vi "Top_Level_Control_1SDI_v00.vi"() -> ()   [LabVIEW 2013]
uses:
  Strict Type Defs/1BS3HD Control GUI HD.ctl
  Strict Type Defs/PII Gains.ctl
  Strict Type Defs/I16 white control.ctl
  Strict Type Defs/Thresh slider.ctl
  Strict Type Defs/Lock or Hold.ctl
  Strict Type Defs/Scan Freq Slider.ctl
  Strict Type Defs/Gains negative horizontal.ctl
  Strict Type Defs/Slider and display.ctl
  Strict Type Defs/theta 1SDI.ctl
  Strict Type Defs/1BS3HD Control GUI EPR.ctl
  Strict Type Defs/1BS3HD Lock Select.ctl
  Strict Type Defs/Scope and Safety.ctl
  Strict Type Defs/Hold All.ctl
  <vilib>/userdefined/High Color/nirio_resource_hc.ctl
  Strict Type Defs/1BS3HD Extras.ctl
  Strict Type Defs/1BS3HD Double control.ctl
  Strict Type Defs/1BS3HD I16 Control.ctl
  <vilib>/FPGAPlugInAG/PXI-7852R/niLvFpga_Open_PXI-7852R.vi
  <vilib>/rvi/interface/common/dynamic/niFpgaDynamicAddResources.vi
  <vilib>/rvi/interface/common/niFpgaWaitOnOcc.vi
  <vilib>/Utility/error.llb/Error Cluster From Error Code.vi
  <vilib>/rvi/errors/niLvFpgaAdjustHostInterfaceError.vi
  <vilib>/FPGAPlugInAG/Dynamic/niLvFpga_Close_Dynamic.vi
  <vilib>/rvi/interface/nirviOpenFPGA/nirviOpenFPGA.xnode
  FPGA Bitfiles/PI-state-4-phase_FPGATarget_3HD1BSFPGAv00_skdKazwPNYA.lvbitx
  <vilib>/rvi/interface/nirviReadWriteControl/nirviReadWriteControl.xnode
  <vilib>/rvi/interface/nirviMethod/nirviMethod.xnode
  <vilib>/rvi/interface/nirviCloseFPGA/nirviCloseFPGA.xnode
  <vilib>/rvi/interface/Simulation/niFpgaSimulationCallBeginRW.vi
  NiFpgaLv.dll
  <vilib>/FPGAPlugInAG/Dynamic/niLvFpga_ReadFifo_Dynamic.vi
  <vilib>/rvi/errors/niLvFpgaMergeErrorWithErrorCode.vi
panel:
  in  "watertank":bool
  out "Water Tank":dbl(slide)=nan scale=-0.3..0.3
  out "Top Loop Count":i32=219749
  in  "stop":bool
  in  "Hold All":T1
  in  "Extra Controls":enum32{"Scope", "Extra Controls", "X-Y Resurge"}(tab)=enum."X-Y Resurge"
  in  "Scope+Safety":T2={"Safety First"={"lim reset"=FALSE, "no limit"=FALSE, "pos slew rate * dt"=240, "neg slew rate * dt"=-240, "Count(Ticks)"=0}, "Scope IPs"={"Trigger Direction"=enum."minus-plus", "Trigger Delay (ms)"=0.0, "Aquisition Rate (kHz)"=4000.0, "Trigger Offset (V)"=0.0, "Scale Offset"={"Scaling"={"Error signal"=1, "Output"=0, "DC Monitor"=1, "Threshold"=1}, "Offset"={"Error Signal"=0, "Output"=0, "DC Monitor"=0, "Threshold"=0}}}}
  in  "Extras 1SDI":T3={"Error Bit Shift "={"EPR BS"=-1, "HD A x"=-3, "HD A p"=-3, "HD B x"=-3, "HD B p"=-3, "HD C x"=-3, "HD C p"=-3}, "I Max value"=200000, "Scan Offset"={"EPR BS"=0.0, "HD A"=1000.0, "HD B"=0.0, "HD C"=0.0}, "Scan Ampl.\n     (mV)"={"EPR BS"=5000.0, "HD A"=5000.0, "HD B"=5000.0, "HD C"=5000.0}, "Scan-PII thresh"={"EPR BS"=100, "Homodyne A"=100, "Homodyne B"=100, "Homodyne C"=100}, "Re-Scan thresh"={"EPR BS"=1, "Homodyne A"=10, "Homodyne B"=1, "Homodyne C"=0}, "Post-Offset"={"HD A x"=0.0, "HD A p"=0.0, "HD B x"=0.0, "HD B p"=0.0, "HD C x"=0.0, "HD C p"=0.0}}
  out "Graph error":errorcluster
  in  "Number of Elements":u32=4095
  in  "1SDI_FPGA_v00":T6="RIO0" caption="RIO Device"
  out "xy HD A":cluster{i16[], i16[]}(graph)
  in  "XY HD 12 ON":bool
  out "xy HD B":cluster{i16[], i16[]}(graph)
  out "xy HD B 2":cluster{i16[], i16[]}(graph)
  in  "XY HD 3 ON":bool
  in  "Scope":T7=TRUE
  out "Scope Graph":cluster{dbl[], dbl[]}[](graph)
  in  "Lock Select":T8
  in  "EPR BS":T9={"Offset Error"=-0.0003389830508474583, "Gain Error"=1, "P Gain"=16, "P Bit Shift"=-4, "I Bit Shift"=-5, "I Gain"=14, "Lock Threshold"=7, "Lock"=FALSE, "Hold"=FALSE, "Scan Frequency"=30, "Scan Bit Shift"=-7, "Gains +/- "=TRUE, "Pre- Offset Error"=0.0077966101694915265} {"Pre- Offset Error" scale=-0.01..0.02 scale format="%#_5f"; "Scan Frequency" scale=1.0..30.0; "I Gain" scale=0.0..50.0; "P Gain" scale=0.0..50.0; "Offset Error" scale=-0.02..0.02 scale format="%#_5f"}
  in  "Homodyne A":T16={"P Gain"=15, "P Bit Shift"=-4, "I Bit Shift"=-6, "I Gain"=19, "Lock Threshold"=19, "Lock"=FALSE, "Hold"=FALSE, "Scan Frequency"=11, "Scan Bit Shift"=-5, "Gains +/- "=TRUE, "Pre- Offset x"=0.008870056497175142, "Pre-Offset p"=0.0011864406779661, "Gain Error x"=3, "Lock Angle"=90.0, "Gain Error p\n\n"=7} {"Lock Angle" min=-90.0 max=90.0 scale=-90.0..90.0 scale format="%#_2g"; "Pre-Offset p" scale=-0.01..0.01 scale format="%#_5f"; "Pre- Offset x" scale=-0.03..0.05 scale format="%#_5f"; "Scan Frequency" scale=1.0..30.0; "I Gain" scale=0.0..50.0; "P Gain" scale=0.0..50.0}
  in  "Homodyne B":T16={"P Gain"=15, "P Bit Shift"=-6, "I Bit Shift"=-7, "I Gain"=21, "Lock Threshold"=16, "Lock"=FALSE, "Hold"=FALSE, "Scan Frequency"=11, "Scan Bit Shift"=-5, "Gains +/- "=TRUE, "Pre- Offset x"=-0.007062146892655368, "Pre-Offset p"=-0.0018644067796610183, "Gain Error x"=2, "Lock Angle"=0.0, "Gain Error p\n\n"=7} {"Lock Angle" min=-90.0 max=90.0 scale=-90.0..90.0 scale format="%#_2g"; "Pre-Offset p" scale=-0.03..0.03 scale format="%#_5f"; "Pre- Offset x" scale=-0.05..0.05 scale format="%#_5f"; "Scan Frequency" scale=1.0..30.0; "I Gain" scale=0.0..50.0; "P Gain" scale=0.0..50.0}
  in  "Homodyne C":T16={"P Gain"=19, "P Bit Shift"=-6, "I Bit Shift"=-7, "I Gain"=17, "Lock Threshold"=16, "Lock"=FALSE, "Hold"=FALSE, "Scan Frequency"=13, "Scan Bit Shift"=-5, "Gains +/- "=TRUE, "Pre- Offset x"=0.01327683615819209, "Pre-Offset p"=0.007627118644067794, "Gain Error x"=2, "Lock Angle"=90.0, "Gain Error p\n\n"=5} {"Lock Angle" min=-90.0 max=90.0 scale=-90.0..90.0 scale format="%#_2g"; "Pre-Offset p" scale=-0.03..0.03 scale format="%#_5f"; "Pre- Offset x" scale=-0.05..0.05 scale format="%#_5f"; "Scan Frequency" scale=1.0..30.0; "I Gain" scale=0.0..50.0; "P Gain" scale=0.0..50.0}
  # "Error Signal"
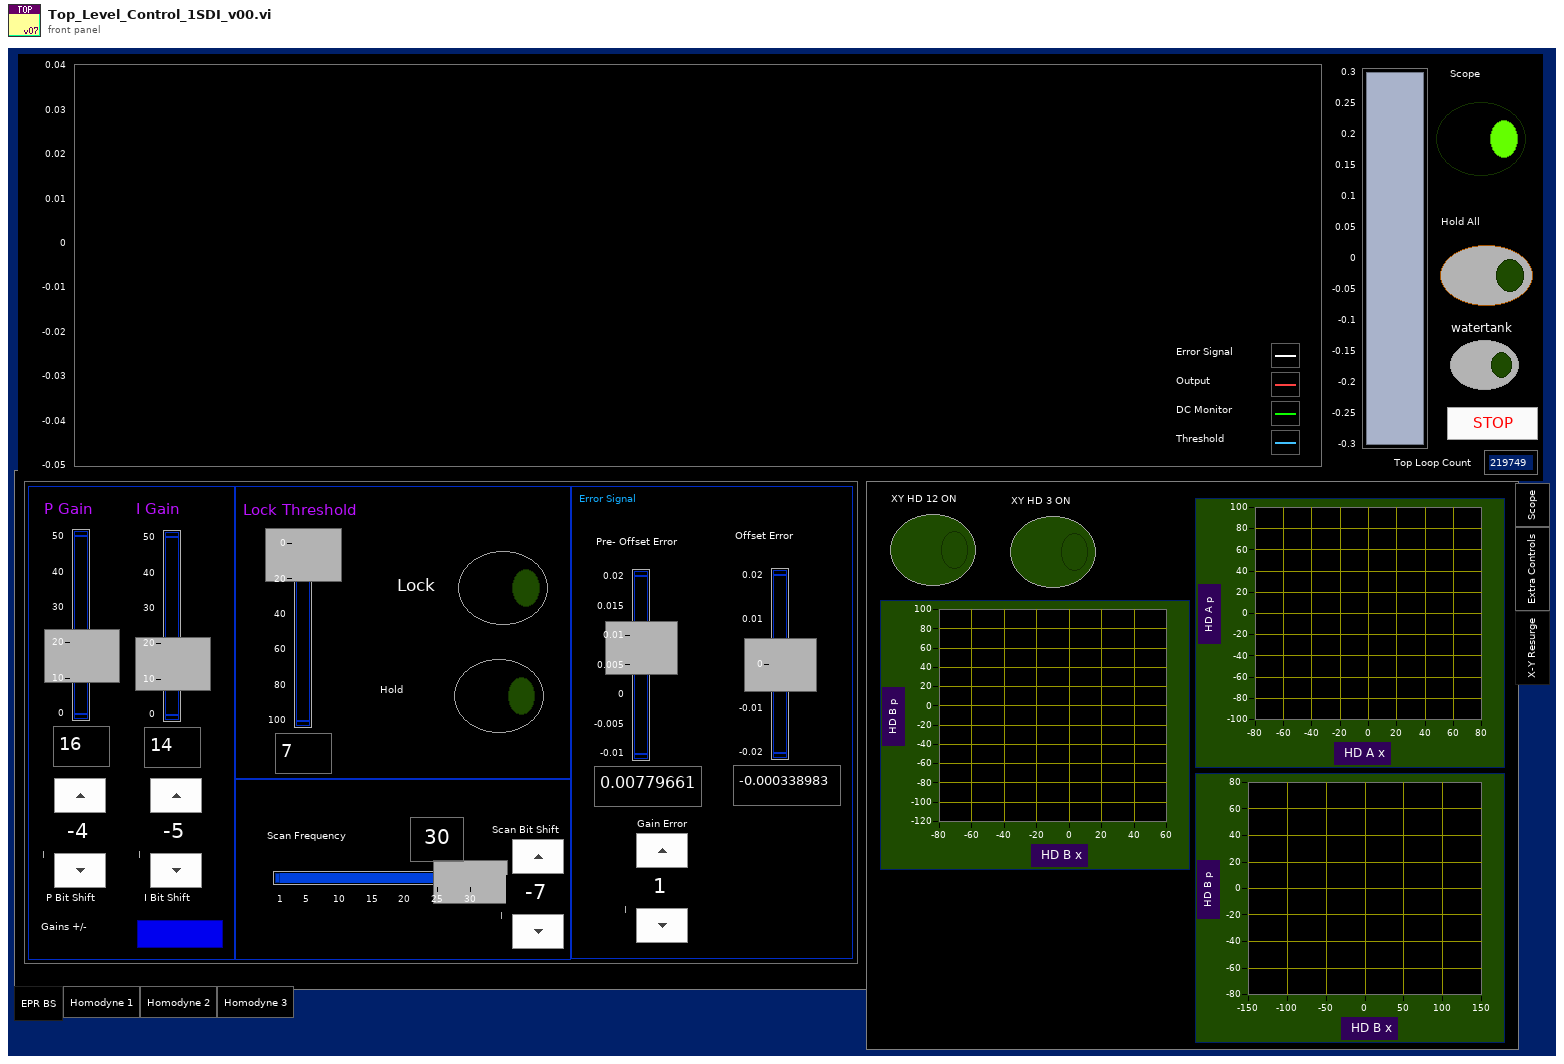
[diagram p1: front panel]
types:
  T1 = typedef "Hold All.ctl" = bool
  T2 = typedef "Scope and Safety.ctl" = cluster{"Safety First":cluster{"lim reset":bool, "no limit":bool, "pos slew rate * dt":i16, "neg slew rate * dt":i16, "Count(Ticks)":u32}, "Scope IPs":cluster{"Trigger Direction":enum8{"either", "minus-plus", "plus-minus"}, "Trigger Delay (ms)":dbl, "Aquisition Rate (kHz)":dbl, "Trigger Offset (V)":dbl, "Scale Offset":cluster{"Scaling":cluster{"Error signal":i16, "Output":i16, "DC Monitor":i16, "Threshold":i16}, "Offset":cluster{"Error Signal":i16, "Output":i16, "DC Monitor":i16, "Threshold":i16}}}}
  T3 = typedef "1BS3HD Extras.ctl" = cluster{"Error Bit Shift ":cluster{"EPR BS":i16, "HD A x":i16, "HD A p":i16, "HD B x":i16, "HD B p":i16, "HD C x":i16, "HD C p":i16}, "I Max value":i32, "Scan Offset":T4, "Scan Ampl.\n     (mV)":T4, "Scan-PII thresh":T5, "Re-Scan thresh":T5, "Post-Offset":cluster{"HD A x":dbl, "HD A p":dbl, "HD B x":dbl, "HD B p":dbl, "HD C x":dbl, "HD C p":dbl}}
  T4 = typedef "1BS3HD Double control.ctl" = cluster{"EPR BS":dbl, "HD A":dbl, "HD B":dbl, "HD C":dbl}
  T5 = typedef "1BS3HD I16 Control.ctl" = cluster{"EPR BS":i16, "Homodyne A":i16, "Homodyne B":i16, "Homodyne C":i16}
  T6 = typedef "nirio_resource_hc.ctl" = tag
  T7 = typedef "Lock or Hold.ctl" = bool
  T8 = typedef "1BS3HD Lock Select.ctl" = enum32{"EPR BS", "Homodyne 1", "Homodyne 2", "Homodyne 3"}
  T9 = typedef "1BS3HD Control GUI EPR.ctl" = cluster{"Offset Error":T10, "Gain Error":T11, "P Gain":T12, "P Bit Shift":T11, "I Bit Shift":T11, "I Gain":T12, "Lock Threshold":T13, "Lock":T7, "Hold":T7, "Scan Frequency":T14, "Scan Bit Shift":T11, "Gains +/- ":T15, "Pre- Offset Error":T10}
  T10 = typedef "Slider and display.ctl" = dbl
  T11 = typedef "I16 white control.ctl" = i16
  T12 = typedef "PII Gains.ctl" = i32
  T13 = typedef "Thresh slider.ctl" = i16
  T14 = typedef "Scan Freq Slider.ctl" = u16
  T15 = typedef "Gains negative horizontal.ctl" = bool
  T16 = typedef "1BS3HD Control GUI HD.ctl" = cluster{"P Gain":T12, "P Bit Shift":T11, "I Bit Shift":T11, "I Gain":T12, "Lock Threshold":T13, "Lock":T7, "Hold":T7, "Scan Frequency":T14, "Scan Bit Shift":T11, "Gains +/- ":T15, "Pre- Offset x":T10, "Pre-Offset p":T10, "Gain Error x":T11, "Lock Angle":T17, "Gain Error p\n\n":T11}
  T17 = typedef "theta 1SDI.ctl" = dbl
  T18 = typedef "1BS3HD Control dummy.ctl" = cluster{"PII In 1":cluster{"Lock":bool, "Hold":bool, "P Gain":i32, "P BS":i16, "I Gain":i32, "I BS":i16, "I2 G":i32, "I2 BS":i16, "Scan Amp":i16, "Scan Off":i16, "Scan FS":u16, "SFS BS":i16, "I Max value":i32, "I2 Max value":i32, "Scope.Offset":i16, "Trigger Direction":enum8{"either", "minus-plus", "plus-minus"}, "Scan-PII thresh":i16}, "PII In 2":cluster{"Lock":bool, "Hold":bool, "P Gain":i32, "P BS":i16, "I Gain":i32, "I BS":i16, "I2 G":i32, "I2 BS":i16, "Scan Amp":i16, "Scan Off":i16, "Scan FS":u16, "SFS BS":i16, "I Max value":i32, "I2 Max value":i32, "Scope.Offset":i16, "Trigger Direction":enum8{"either", "minus-plus", "plus-minus"}, "Scan-PII thresh":i16}, "PII In 3":cluster{"Lock":bool, "Hold":bool, "P Gain":i32, "P BS":i16, "I Gain":i32, "I BS":i16, "I2 G":i32, "I2 BS":i16, "Scan Amp":i16, "Scan Off":i16, "Scan FS":u16, "SFS BS":i16, "I Max value":i32, "I2 Max value":i32, "Scope.Offset":i16, "Trigger Direction":enum8{"either", "minus-plus", "plus-minus"}, "Scan-PII thresh":i16}, "Error scale":cluster{"Pre-Offset":cluster{"Pre-Offset 1":i16, "Pre-Offset 2":i16, "Pre-Offset 3":i16, "Pre-Offset 4":i16, "Pre-Offset 5":i16, "Pre-Offset 6":i16, "Pre-Offset 7":i16}, "Post-Offset ":cluster{"Offset 1":i16, "Offset 2":i16, "Offset 3":i16, "Offset 4":i16, "Offset 5":i16, "Offset 6":i16, "Offset 7":i16}, "Gains":cluster{"Gain 1":i16, "Gain 2":i16, "Gain 3":i16, "Gain 4":i16, "Gain 5":i16, "Gain 7":i16, "Gain 6":i16}, "Bit Shifts":cluster{"Bit Shift 1":i16, "Bit Shift 2":i16, "Bit Shift 3":i16, "Bit Shift 4":i16, "Bit Shift 5":i16, "Bit Shift 6":i16, "Bit Shift 7":i16}}, "Lock Thresh":cluster{"EPR":i16, "HD A":i16, "HD B":i16, "HD C":i16}, "Re-Scan Thresh":cluster{"EPR":i16, "HD A":i16, "HD B":i16, "HD C":i16}, "Theta":cluster{"HD A Sin Theta":i32, "HD A Cos Theta":i32, "HD B Sin Theta":i32, "HD B Cos Theta":i32, "HD C Cos Theta":i32, "HD C Sin Theta":i32}, "Safety First":cluster{"lim reset":bool, "no limit":bool, "pos slew rate * dt":i16, "neg slew rate * dt":i16, "Hold All":bool, "Count(Ticks)":u32}, "PII In 4":cluster{"Lock":bool, "Hold":bool, "P Gain":i32, "P BS":i16, "I Gain":i32, "I BS":i16, "I2 G":i32, "I2 BS":i16, "Scan Amp":i16, "Scan Off":i16, "Scan FS":u16, "SFS BS":i16, "I Max value":i32, "I2 Max value":i32, "Scope.Offset":i16, "Trigger Direction":enum8{"either", "minus-plus", "plus-minus"}, "Scan-PII thresh":i16}}
  T19 = cluster{"Trigger Direction":enum8{"either", "minus-plus", "plus-minus"}, "Delay":u32, "Aquisition Rate (Ticks)":u32, "Offset":i16, "Channel":i32, "Channel Selector":cluster{"Channel 1":i32, "Channel 2":i32, "Channel 3":i32, "Channel 4":i32}}
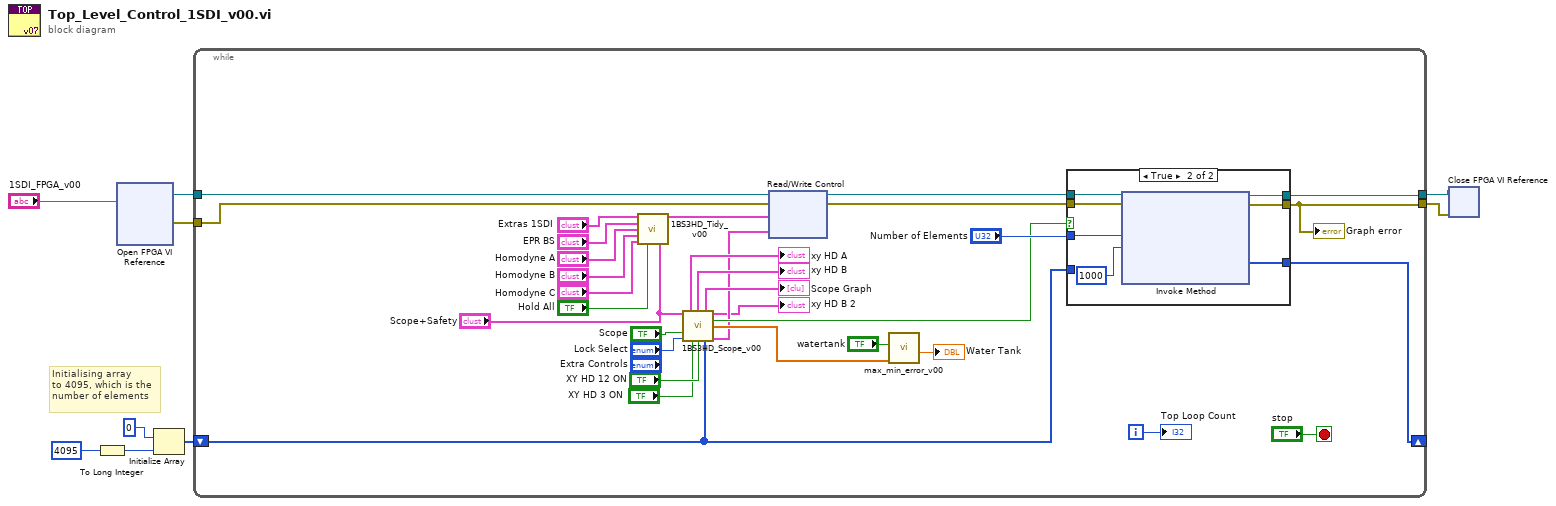
[diagram p0: block diagram]
diagram:
  # "Initialising array\nto 4095, which is the\nnumber of elements"
  n1 = To Long Integer(number=4095) -> (32bit integer=w9:i32)
  n2 = xnode "Open FPGA VI Reference"("resource name"="1SDI_FPGA_v00") -> ("FPGA VI Reference Out"=w5:refnum<k20>, "error out"=w4:errorcluster)  [unwired: 1 in]
  n3 = Initialize Array(u64 0 ("element"), w9) -> (w1:u64[])
  n4 = while {
    tunnel: w5 -> [w15]
    tunnel: w4 -> [w14]
    tunnel: [w38] -> w3
    tunnel: [w37] -> w2
    shift-right: [w35] -> _
    shift-left: w1 -> [w34]
    i -> [w40]
    stop <- "stop" stop-if-true
    n5 = call "1BS3HD_Tidy_v00.vi"("Extras 1SDI"="Extras 1SDI", "EPR BS"="EPR BS", "Homodyne A"="Homodyne A", "Homodyne B"="Homodyne B", "Homodyne C"="Homodyne C", "Hold All"="Hold All", "Scope+Safety"="Scope+Safety") -> ("1SDI Control"=w16:T18)  [unwired: 8 in]
    n6 = call "1BS3HD_Scope_v00.vi"("Scope+Safety"="Scope+Safety", "Scope"="Scope", "Lock Select"="Lock Select", "XY HD 3 ON"="XY HD 3 ON", "XY HD 12 ON"="XY HD 12 ON", "1SDI Data"=w34) -> ("xy HD 1"=→"xy HD A":cluster{i16[], i16[]}, "xy HD 2"=→"xy HD B":cluster{i16[], i16[]}, "Scope OP 1SDI"=→"Scope Graph":cluster{dbl[], dbl[]}[], "xy HD 3"=→"xy HD B 2":cluster{i16[], i16[]}, "Scope 1SDI ON"=w31:bool, "error"=w27:dbl[], "Scope 1SDI FPGA"=w19:T19)  [unwired: 3 in]
    n7 = xnode "Read/Write Control"("FPGA VI Reference In"=w15, "error in"=w14, "Control"=w16, "Scope"=w19) -> ("FPGA VI Reference Out"=w24:refnum<k20>, "error out"=w23:errorcluster)
    n8 = call "max_min_error_v00.vi"("Array"=w27, "maxmin"="watertank") -> ("x+y"=→"Water Tank":dbl)  [unwired: 7 in, 2 out]
    n9 = case shown="True" w31 {
      tunnel: w23 -> [w44 w51]
      tunnel: [w44 w50] -> w37
      tunnel: w24 -> [w43 w49]
      tunnel: [w43 w48] -> w38
      tunnel: [w42 w47] -> w35
      tunnel: w34 -> [w42 _]
      tunnel: "Number of Elements" -> [_ w45]
      frame False {
      }
      frame True {
        n10 = xnode "Invoke Method"("FPGA VI Reference In"=w49, "error in"=w51, "Number of Elements"=w45, "Timeout (ms)"=1000) -> ("FPGA VI Reference Out"=w48:refnum<k20>, "error out"=w50:errorcluster, "Data"=w47:u64[])  [unwired: 1 out]
      }
    }
    "Graph error" <- w37
    "Top Loop Count" <- w40
  }
  n11 = xnode "Close FPGA VI Reference"("FPGA VI Reference In"=w3, "error in"=w2) -> ()  [unwired: 1 out]
